vi "connect_password.vi"(8 "error in (no error)":errorcluster, 9 "Connection Name":string, 10 "Password":T1, 11 "Connection Info.":T2={"Remote"="", "Username"="", "Port (22)"=22}) -> (0 "error out":errorcluster, 2 "isSftpConnected":bool, 3 "Return String":string)   [LabVIEW 2017, in "LabSFTP.lvlib"]
doc: "<License>This software is distributed under the BSD 3-Clause License. For the full license please see license.txt or visit www.labvolution.com/license</License>"
uses:
  LabSFTP.lvlib
  Connection Info..cluster.ctl
  Password..cluster.ctl
  FGV State..enum.ctl
  C:/Users/OCT/Downloads/LabSSH-Library-2015/LabSSH Library/References/LabSFTP.dll
  Downloads/LabSSH-Library-2015/LabSSH Library/References/LabSFTP.dll
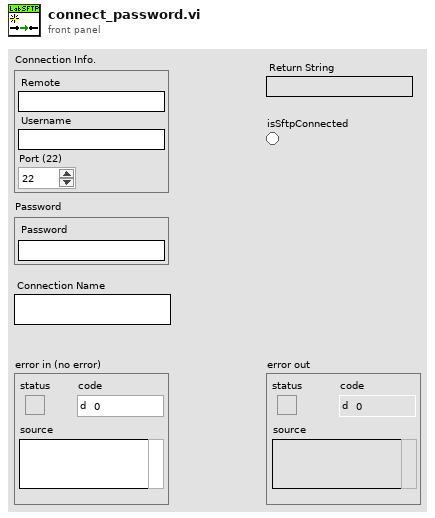
[diagram p1: front panel]
types:
  T1 = typedef "LabSFTP.lvlib/Password..cluster.ctl" = cluster{"Password":string}
  T2 = typedef "LabSFTP.lvlib/Connection Info..cluster.ctl" = cluster{"Remote":string, "Username":string, "Port (22)":i32}
  T3 = typedef "LabSFTP.lvlib/FGV State..enum.ctl" = enum16{"GET", "SET"}
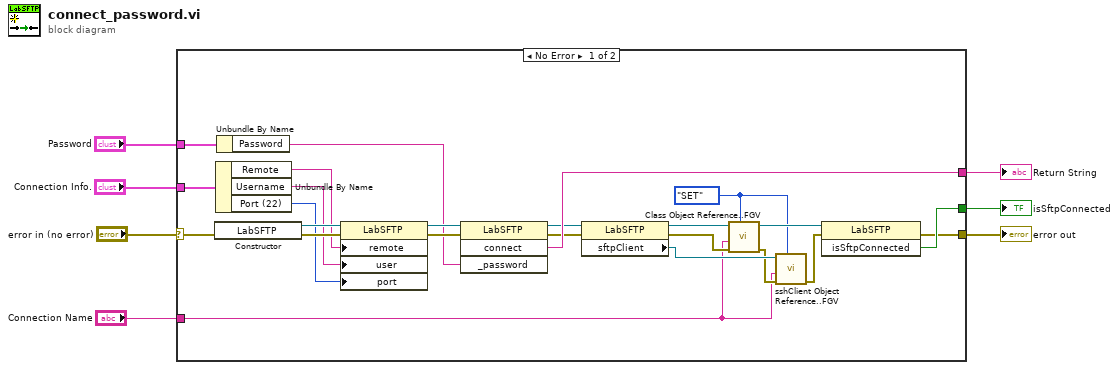
[diagram p0: block diagram]
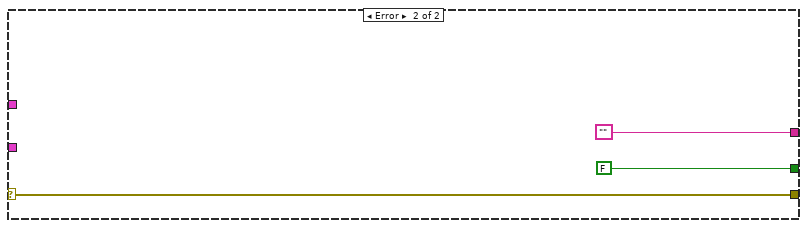
[diagram p2: hidden frame]
diagram:
  n1 = case shown="No Error" "error in (no error)" {
    selector: "error in (no error)" -> [w28 w34]
    tunnel: [w31 FALSE ("isSshConnected")] -> w7
    tunnel: "Password" -> [w30 _]
    tunnel: [w29 ""] -> w6
    tunnel: "Connection Info." -> [w22 _]
    tunnel: [w17 w34] -> w3
    tunnel: "Connection Name" -> [w8 _]
    frame No Error {
      w13 = FGV_State..enum."SET" ("FGV State")
      n2 = constructor class="LabSFTP" ("Constructor Node")(error in=w28) -> (reference out=w27:refnum<k24>, error out=w23:errorcluster)  [unwired: 2 in, 1 out]
      n3 = Unbundle By Name(w22) -> ("Remote"=w21:string, "Username"=w20:string, "Port (22)"=w19:i32)
      n4 = Unbundle By Name(w30) -> ("Password"=w9:string)
      n5 = property on="Property Node" class="LabSFTP"(reference=w27, error in=w23, "remote"=w21, "user"=w20, "port"=w19) -> (reference out=w26:refnum<k24>, error out=w24:errorcluster)
      n6 = invoke on="Invoke Node" class="LabSFTP" method="connect"(reference=w26, error in=w24, "_password"=w9) -> (reference out=w18:refnum<k24>, error out=w25:errorcluster, "connect"=w29:string)  [unwired: 1 in, 1 out]
      n7 = property class="LabSFTP"(reference=w18, error in=w25) -> (reference out=w16:refnum<k24>, error out=w14:errorcluster, "sftpClient"=w11:refnum<k24>)
      n8 = call "Class Object Reference..FGV.vi"("FGV State"=w13, "error in (no error)"=w14, "Connection Name"=w8, "LabSFTP ref in"=w16) -> ("error out"=w10:errorcluster, "LabSFTP ref out"=w15:refnum<k24>)  [unwired: 6 in]
      n9 = call "sshClient Object Reference..FGV.vi"("FGV State"=w13, "error in (no error)"=w10, "Connection Name"=w8, "sftpClient ref in"=w11) -> ("error out"=w12:errorcluster)  [unwired: 6 in, 1 out]
      n10 = invoke on="Invoke Node" class="LabSFTP" method="isSftpConnected"(reference=w15, error in=w12) -> (error out=w17:errorcluster, "isSftpConnected"=w31:bool)  [unwired: 1 in, 1 out]
    }
    frame Error {
    }
  }
  "error out" <- w3
  "isSftpConnected" <- w7
  "Return String" <- w6
